vi "Set Tuner Gain Mode.vi"(8 "error in (no error)":errorcluster, 10 "Tuner Gain Mode":T1 items=["Automatic", "Manual"], 11 "RTL-SDR in":refnum<class "Session.lvclass">) -> (0 "error out":errorcluster, 3 "RTL-SDR out":refnum<class "Session.lvclass">)   [LabVIEW 2020, in "RTL-SDR.lvlib" / "Session.lvclass"]
uses:
  Session.lvclass
  C:/dev/IlluminatedG/lv-rtl-sdr/lib/librtlsdr.dll
  Gain Mode.ctl
  RTL-SDR.lvlib
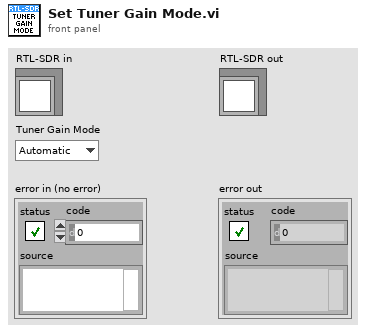
[diagram p1: front panel]
types:
  T1 = typedef "RTL-SDR.lvlib/Gain Mode.ctl" = i32
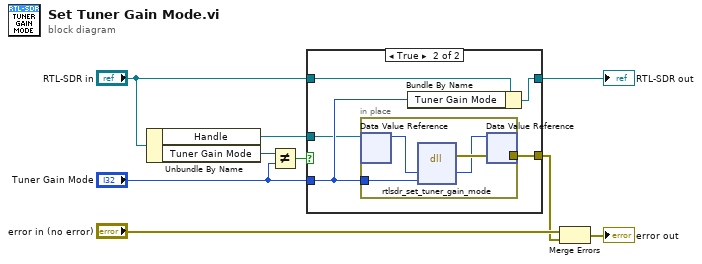
[diagram p0: block diagram]
diagram:
  n1 = Unbundle By Name("RTL-SDR in") -> ("Handle"=w6:refnum<data-value>, "Tuner Gain Mode"=w8:T1)
  n2 = Not Equal?(x=w8, y="Tuner Gain Mode") -> (x != y?=w7:bool)
  n3 = case shown="True" w7 {
    tunnel: w6 -> [_ w11]
    tunnel: "Tuner Gain Mode" -> [_ w13]
    tunnel: [_ w15] -> w3
    tunnel: "RTL-SDR in" -> [w10 w14]
    tunnel: [w10 w12] -> w1
    frame False {
    }
    frame True {
      n4 = in-place {
        in-place-border: [w19] -> w15
        in-place-border: w13 -> [w18]
        n5 = in-place-dvr #1(w11) -> (w17:u64)  [unwired: 1 out]
        n6 = dll-call lib="C:/dev/IlluminatedG/lv-rtl-sdr/lib/librtlsdr.dll" fn="rtlsdr_set_tuner_gain_mode"("dev"=w17, "manual"=w18) -> (error out=w19:errorcluster, "dev"=w16:u64)  [unwired: 5 in, 1 out]
        n7 = in-place-dvr #1(w16) -> ()  [unwired: 2 out]
      }
      n8 = Bundle By Name(cluster=w14, "Tuner Gain Mode"=w13) -> (w12:refnum<class "Session.lvclass">)
    }
  }
  "RTL-SDR out" <- w1
  n9 = Merge Errors("error in (no error)", w3) -> (→"error out":errorcluster)
